vi "SignalProcessing.vi"(1 "E2S":dbl[](array[numeric]), 2 "E3S":dbl[](array[numeric]), 3 "E4S":dbl[](array[numeric]), 4 "E5S":dbl[](array[numeric]), 5 "E6S":dbl[](array[numeric]), 6 "E7S":dbl[](array[numeric]), 7 "E9S":dbl[](array[numeric]), 9 "E8S":dbl[](array[numeric]), 10 "E1S":dbl[](array[numeric]), 11 "Corte Alto":dbl(knob) scale=10.0..50.0, 13 "Muestreo":dbl) -> (12 "X1":dynamicdata(graph), 14 "X2":dynamicdata(graph), 16 "X6":dynamicdata(graph), 18 "X3":dynamicdata(graph), 20 "X4":dynamicdata(graph), 21 "X8":dynamicdata(graph), 22 "X5":dynamicdata(graph), 23 "X7":dynamicdata(graph), 24 "X9":dynamicdata(graph))   [LabVIEW 2021]
uses:
  <vilib>/Analysis/3filter.llb/Filter Passband Type.ctl
  <vilib>/Analysis/3filter.llb/Butterworth Filter (DBL).vi
  <vilib>/Analysis/NI_AALBase.lvlib
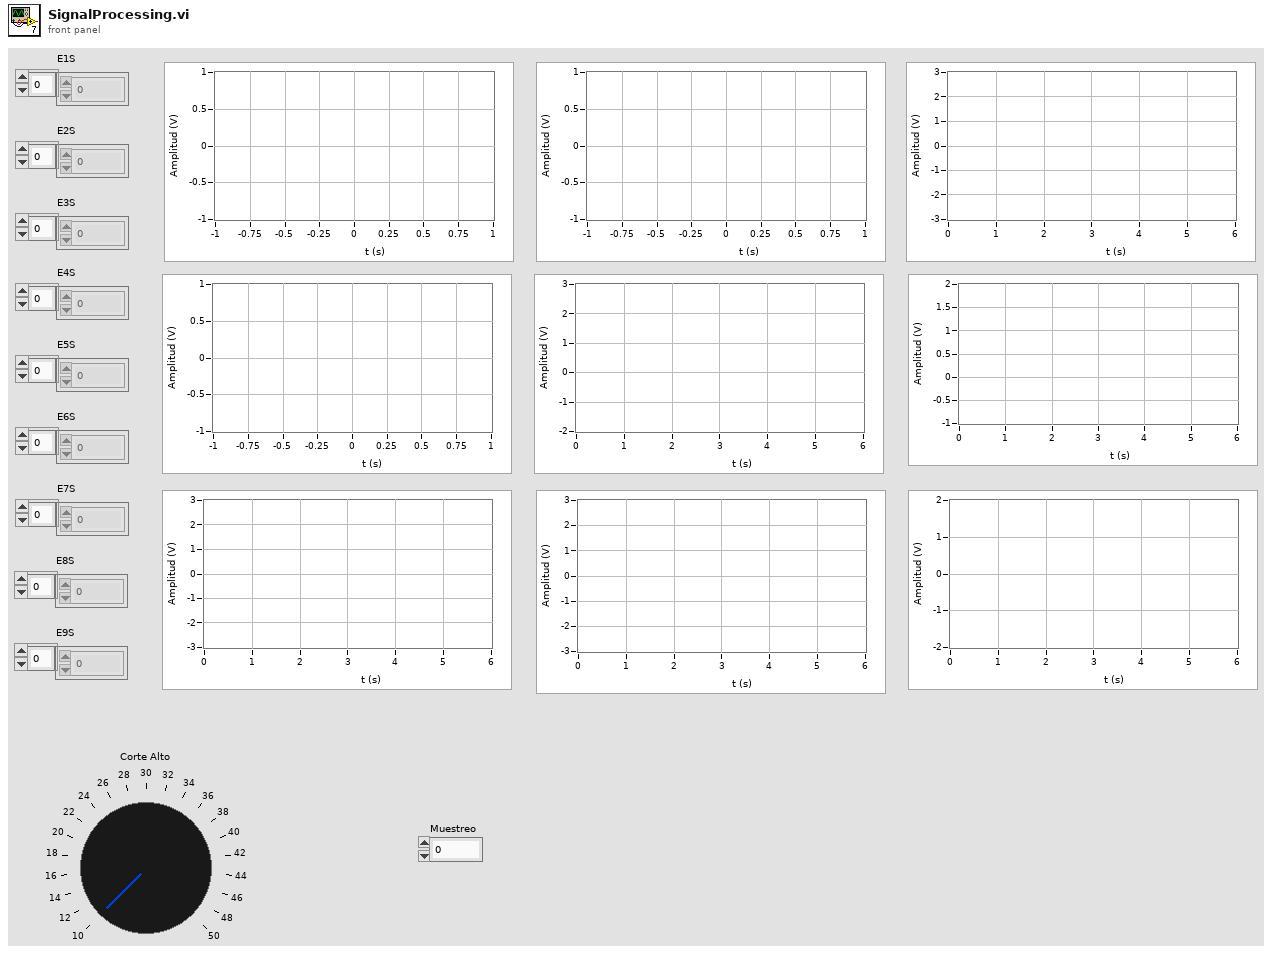
[diagram p1: front panel]
types:
  T1 = typedef "NI_AALBase.lvlib/Filter Passband Type.ctl" = enum32{"Lowpass", "Highpass", "Bandpass", "Bandstop"}
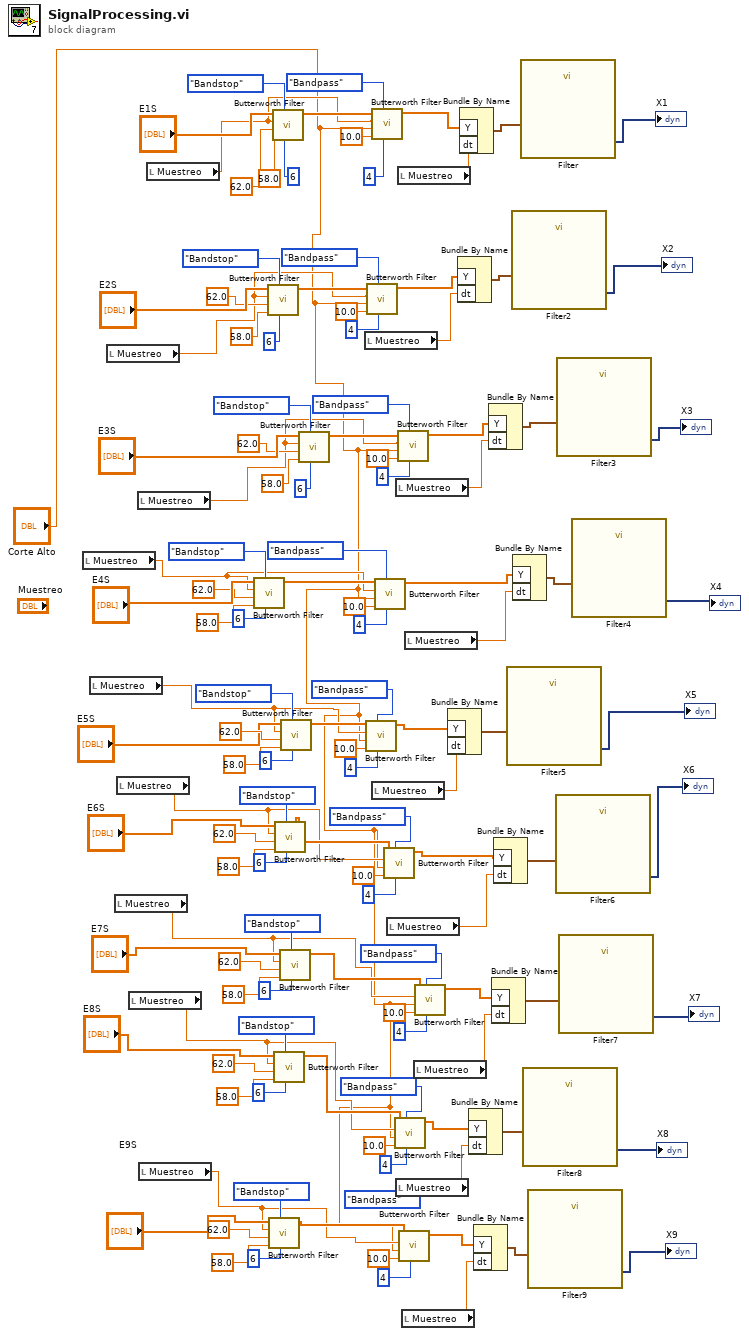
[diagram p0: block diagram]
diagram:
  (unwired) Filter_Passband_Type."Bandpass" ("filter type")
  n1 = local read "Muestreo"() -> (w75:dbl)
  n2 = local read "Muestreo"() -> (w64:dbl)
  n3 = local read "Muestreo"() -> (w78:dbl)
  n4 = local read "Muestreo"() -> (w33:dbl)
  n5 = local read "Muestreo"() -> (w34:dbl)
  n6 = local read "Muestreo"() -> (w20:dbl)
  n7 = local read "Muestreo"() -> (w77:dbl)
  n8 = local read "Muestreo"() -> (w8:dbl)
  n9 = local read "Muestreo"() -> (w120:dbl)
  n10 = call-poly <vilib>:"Butterworth Filter.vi"("order"=6, "filter type"=Filter_Passband_Type."Bandstop", "low cutoff freq: fl"=58.0, "high cutoff freq: fh"=62.0, "sampling freq: fs"=w75, "X"="E4S") -> ("Filtered X"=w87:dbl[])  [unwired: 2 in, 1 out]
  n11 = call-poly <vilib>:"Butterworth Filter.vi"("order"=6, "filter type"=Filter_Passband_Type."Bandstop", "low cutoff freq: fl"=58.0, "high cutoff freq: fh"=62.0, "sampling freq: fs"=w78, "X"="E2S") -> ("Filtered X"=w114:dbl[])  [unwired: 2 in, 1 out]
  n12 = call-poly <vilib>:"Butterworth Filter.vi"("order"=6, "filter type"=Filter_Passband_Type."Bandstop", "low cutoff freq: fl"=58.0, "high cutoff freq: fh"=62.0, "sampling freq: fs"=w8, "X"="E9S") -> ("Filtered X"=w9:dbl[])  [unwired: 2 in, 1 out]
  n13 = call-poly <vilib>:"Butterworth Filter.vi"("order"=6, "filter type"=Filter_Passband_Type."Bandstop", "low cutoff freq: fl"=58.0, "high cutoff freq: fh"=62.0, "sampling freq: fs"=w120, "X"="E1S") -> ("Filtered X"=w121:dbl[])  [unwired: 2 in, 1 out]
  n14 = call-poly <vilib>:"Butterworth Filter.vi"("order"=6, "filter type"=Filter_Passband_Type."Bandstop", "low cutoff freq: fl"=58.0, "high cutoff freq: fh"=62.0, "sampling freq: fs"=w20, "X"="E8S") -> ("Filtered X"=w21:dbl[])  [unwired: 2 in, 1 out]
  n15 = call-poly <vilib>:"Butterworth Filter.vi"("order"=6, "filter type"=Filter_Passband_Type."Bandstop", "low cutoff freq: fl"=58.0, "high cutoff freq: fh"=62.0, "sampling freq: fs"=w34, "X"="E6S") -> ("Filtered X"=w48:dbl[])  [unwired: 2 in, 1 out]
  n16 = call-poly <vilib>:"Butterworth Filter.vi"("order"=6, "filter type"=Filter_Passband_Type."Bandstop", "low cutoff freq: fl"=58.0, "high cutoff freq: fh"=62.0, "sampling freq: fs"=w33, "X"="E7S") -> ("Filtered X"=w35:dbl[])  [unwired: 2 in, 1 out]
  n17 = call-poly <vilib>:"Butterworth Filter.vi"("order"=6, "filter type"=Filter_Passband_Type."Bandstop", "low cutoff freq: fl"=58.0, "high cutoff freq: fh"=62.0, "sampling freq: fs"=w64, "X"="E5S") -> ("Filtered X"=w65:dbl[])  [unwired: 2 in, 1 out]
  n18 = call-poly <vilib>:"Butterworth Filter.vi"("order"=6, "filter type"=Filter_Passband_Type."Bandstop", "low cutoff freq: fl"=58.0, "high cutoff freq: fh"=62.0, "sampling freq: fs"=w77, "X"="E3S") -> ("Filtered X"=w104:dbl[])  [unwired: 2 in, 1 out]
  n19 = local read "Muestreo"() -> (w109:dbl)
  n20 = call-poly <vilib>:"Butterworth Filter.vi"("order"=4, "filter type"=Filter_Passband_Type."Bandpass", "low cutoff freq: fl"=10.0, "high cutoff freq: fh"="Corte Alto", "sampling freq: fs"=w64, "X"=w65) -> ("Filtered X"=w60:dbl[])  [unwired: 2 in, 1 out]
  n21 = call-poly <vilib>:"Butterworth Filter.vi"("order"=4, "filter type"=Filter_Passband_Type."Bandpass", "low cutoff freq: fl"=10.0, "high cutoff freq: fh"="Corte Alto", "sampling freq: fs"=w78, "X"=w114) -> ("Filtered X"=w110:dbl[])  [unwired: 2 in, 1 out]
  n22 = call-poly <vilib>:"Butterworth Filter.vi"("order"=4, "filter type"=Filter_Passband_Type."Bandpass", "low cutoff freq: fl"=10.0, "high cutoff freq: fh"="Corte Alto", "sampling freq: fs"=w120, "X"=w121) -> ("Filtered X"=w95:dbl[])  [unwired: 2 in, 1 out]
  n23 = local read "Muestreo"() -> (w59:dbl)
  n24 = call-poly <vilib>:"Butterworth Filter.vi"("order"=4, "filter type"=Filter_Passband_Type."Bandpass", "low cutoff freq: fl"=10.0, "high cutoff freq: fh"="Corte Alto", "sampling freq: fs"=w75, "X"=w87) -> ("Filtered X"=w84:dbl[])  [unwired: 2 in, 1 out]
  n25 = call-poly <vilib>:"Butterworth Filter.vi"("order"=4, "filter type"=Filter_Passband_Type."Bandpass", "low cutoff freq: fl"=10.0, "high cutoff freq: fh"="Corte Alto", "sampling freq: fs"=w34, "X"=w48) -> ("Filtered X"=w47:dbl[])  [unwired: 2 in, 1 out]
  n26 = local read "Muestreo"() -> (w46:dbl)
  n27 = call-poly <vilib>:"Butterworth Filter.vi"("order"=4, "filter type"=Filter_Passband_Type."Bandpass", "low cutoff freq: fl"=10.0, "high cutoff freq: fh"="Corte Alto", "sampling freq: fs"=w20, "X"=w21) -> ("Filtered X"=w19:dbl[])  [unwired: 2 in, 1 out]
  n28 = local read "Muestreo"() -> (w100:dbl)
  n29 = local read "Muestreo"() -> (w18:dbl)
  n30 = local read "Muestreo"() -> (w116:dbl)
  n31 = call-poly <vilib>:"Butterworth Filter.vi"("order"=4, "filter type"=Filter_Passband_Type."Bandpass", "low cutoff freq: fl"=10.0, "high cutoff freq: fh"="Corte Alto", "sampling freq: fs"=w77, "X"=w104) -> ("Filtered X"=w101:dbl[])  [unwired: 2 in, 1 out]
  n32 = call-poly <vilib>:"Butterworth Filter.vi"("order"=4, "low cutoff freq: fl"=10.0, "high cutoff freq: fh"="Corte Alto", "sampling freq: fs"=w8, "X"=w9) -> ("Filtered X"=w4:dbl[])  [unwired: 3 in, 1 out]
  n33 = local read "Muestreo"() -> (w3:dbl)
  n34 = local read "Muestreo"() -> (w73:dbl)
  n35 = local read "Muestreo"() -> (w31:dbl)
  n36 = call-poly <vilib>:"Butterworth Filter.vi"("order"=4, "filter type"=Filter_Passband_Type."Bandpass", "low cutoff freq: fl"=10.0, "high cutoff freq: fh"="Corte Alto", "sampling freq: fs"=w33, "X"=w35) -> ("Filtered X"=w32:dbl[])  [unwired: 2 in, 1 out]
  n37 = Bundle By Name("Y"=w60, "dt"=w59) -> (w58:waveform(dbl))  [unwired: 1 in]
  n38 = Bundle By Name("Y"=w110, "dt"=w109) -> (w92:waveform(dbl))  [unwired: 1 in]
  n39 = Bundle By Name("Y"=w95, "dt"=w116) -> (w94:waveform(dbl))  [unwired: 1 in]
  n40 = Bundle By Name("Y"=w19, "dt"=w18) -> (w17:waveform(dbl))  [unwired: 1 in]
  n41 = Bundle By Name("Y"=w4, "dt"=w3) -> (w2:waveform(dbl))  [unwired: 1 in]
  n42 = Bundle By Name("Y"=w101, "dt"=w100) -> (w90:waveform(dbl))  [unwired: 1 in]
  n43 = Bundle By Name("Y"=w32, "dt"=w31) -> (w30:waveform(dbl))  [unwired: 1 in]
  n44 = Bundle By Name("Y"=w47, "dt"=w46) -> (w45:waveform(dbl))  [unwired: 1 in]
  n45 = call "Filter5"("Signal"=w58) -> ("Filtered Signal"=→"X5":dynamicdata)  [unwired: 9 in, 1 out]
  n46 = call "Filter2"("Signal"=w92) -> ("Filtered Signal"=→"X2":dynamicdata)  [unwired: 9 in, 1 out]
  n47 = Bundle By Name("Y"=w84, "dt"=w73) -> (w72:waveform(dbl))  [unwired: 1 in]
  n48 = call "Filter"("Signal"=w94) -> ("Filtered Signal"=→"X1":dynamicdata)  [unwired: 9 in, 1 out]
  n49 = call "Filter8"("Signal"=w17) -> ("Filtered Signal"=→"X8":dynamicdata)  [unwired: 9 in, 1 out]
  n50 = call "Filter9"("Signal"=w2) -> ("Filtered Signal"=→"X9":dynamicdata)  [unwired: 9 in, 1 out]
  n51 = call "Filter6"("Signal"=w45) -> ("Filtered Signal"=→"X6":dynamicdata)  [unwired: 9 in, 1 out]
  n52 = call "Filter3"("Signal"=w90) -> ("Filtered Signal"=→"X3":dynamicdata)  [unwired: 9 in, 1 out]
  n53 = call "Filter7"("Signal"=w30) -> ("Filtered Signal"=→"X7":dynamicdata)  [unwired: 9 in, 1 out]
  n54 = call "Filter4"("Signal"=w72) -> ("Filtered Signal"=→"X4":dynamicdata)  [unwired: 9 in, 1 out]
